vi "Read Valid Messages.vi"(8 "error in (no error)":errorcluster, 11 "Temperature Controller in":refnum<class "Temperature Controller.lvclass">) -> (0 "error out":errorcluster, 2 "Valid Messages":string[](array[string]), 3 "Temperature Controller out":refnum<class "Temperature Controller.lvclass">)   [LabVIEW 2020, in "RxnRover.lvlib" / "Temperature Controller.lvclass"]
uses:
  Temperature Controller.lvclass
  Temperature Controller.lvclass/Temperature Controller.ctl
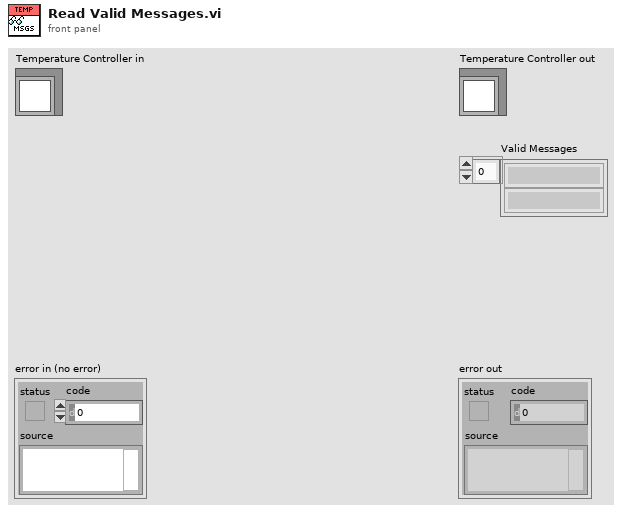
[diagram p1: front panel]
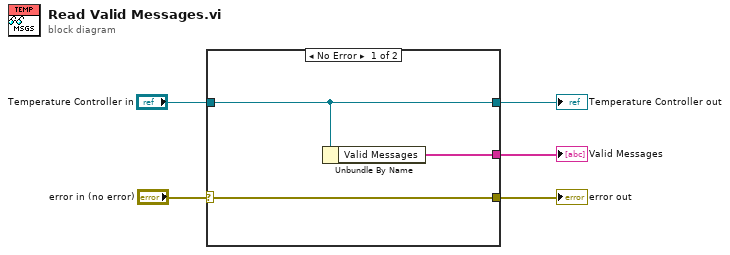
[diagram p0: block diagram]
diagram:
  n1 = case shown="No Error" "error in (no error)" {
    selector: "error in (no error)" -> [w6 w10]
    tunnel: "Temperature Controller in" -> [w7 w9]
    tunnel: [w8 _] -> w4
    tunnel: [w7 w9] -> w3
    tunnel: [w6 w10] -> w1
    frame No Error {
      n2 = Unbundle By Name(w7) -> ("Valid Messages"=w8:string[])
    }
    frame Error {
    }
  }
  "error out" <- w1
  "Temperature Controller out" <- w3
  "Valid Messages" <- w4
